vi "System@IncludeModule__Parameter.vi"(1 "ParamterIn":string) -> (0 "ParamterOut":string)   [LabVIEW 2020]
uses:
  MainFrame/Global.vi
panel:
  in  "Debug":string(combo)
  in  "Module":string(combo)
  in  "Confirm":bool
  # "System@IncludeModule $Module(,Debug)\nModule Directory is at MainPath\\ExternalModules\\$Module"
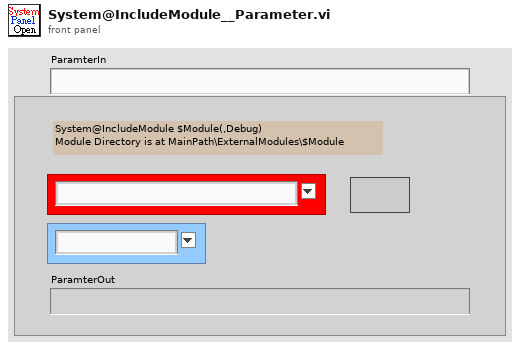
[diagram p1: front panel]
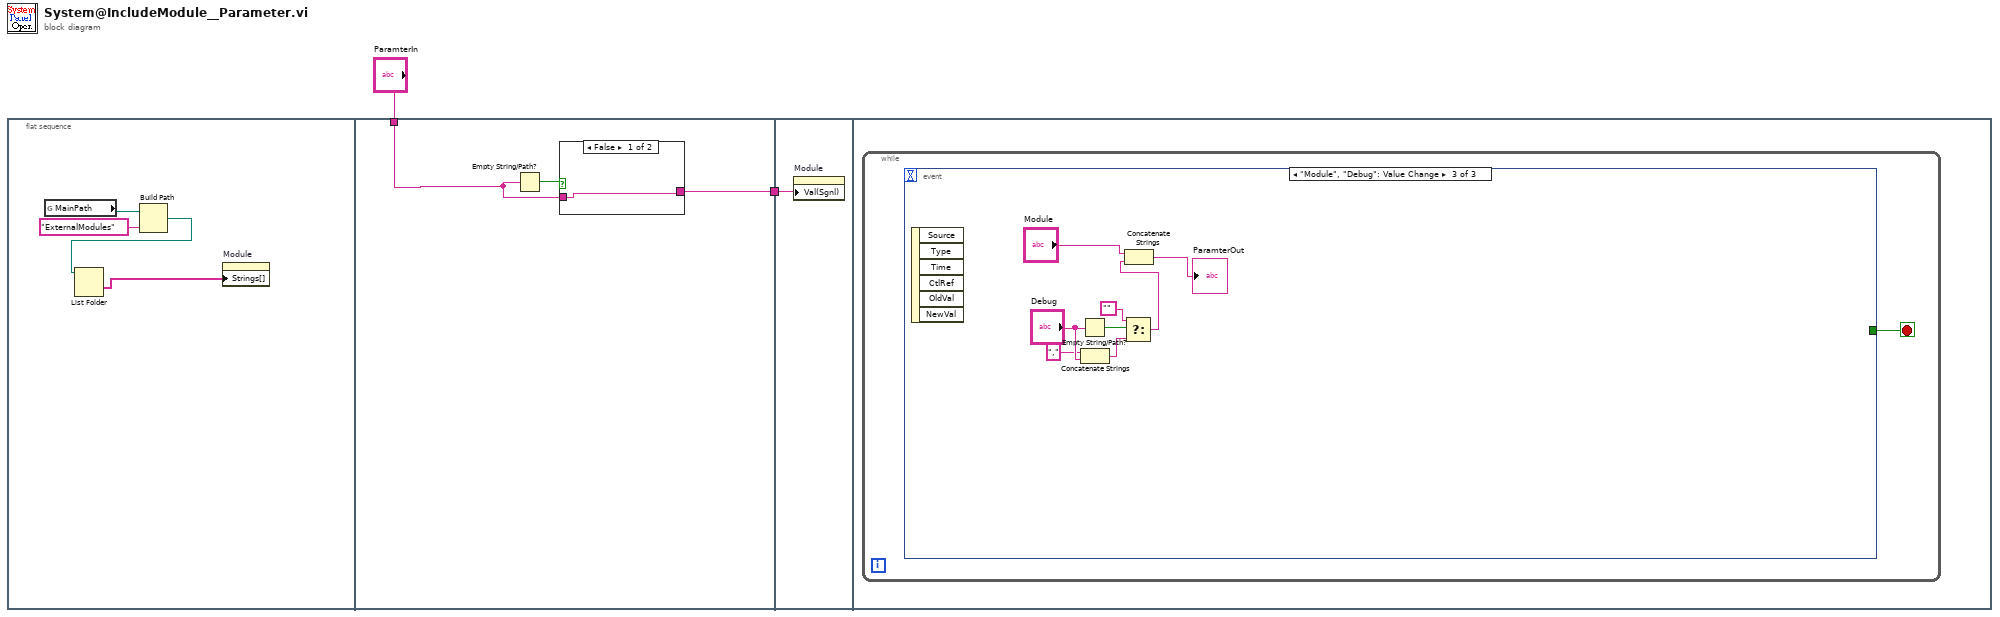
[diagram p0: block diagram]
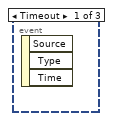
[diagram p3: hidden frame]
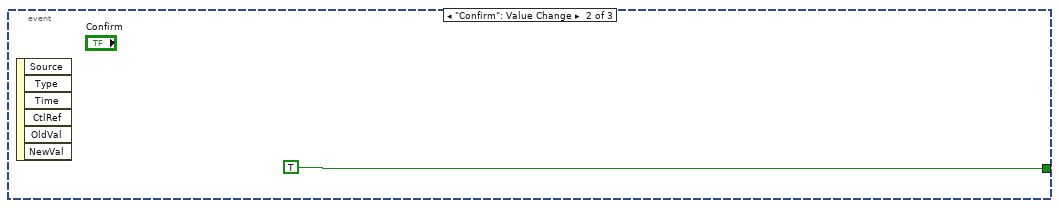
[diagram p4: hidden frame]
diagram:
  n1 = flat-sequence {
    tunnel: "ParamterIn" -> [w7]
    tunnel: [w8] -> w1
    tunnel: w1 -> [w12]
    frame #0 {
      n2 = global read "Global.vi" "MainPath"() -> (w6:path)
      n3 = Build Path(base path=w6, name or relative path="ExternalModules") -> (appended path=w4:path)
      n4 = List Folder(path=w4) -> (folder names=w3:string[])  [unwired: 3 in, 3 out]
      n5 = property on="Module" class="CmbBox"("Strings[]"=w3) -> ()  [unwired: 2 in, 2 out]
    }
    frame #1 {
      n6 = Empty String/Path?(string/path=w7) -> (empty?=w9:bool)
      n7 = case shown="False" w9 {
        tunnel: w7 -> [w10 w11]
        tunnel: [w10 w11] -> w8
        frame False {
        }
        frame True {
        }
      }
    }
    frame #2 {
      n8 = property on="Module" class="CmbBox"("Val(Sgnl)"=w12) -> ()  [unwired: 2 in, 2 out]
    }
    frame #3 {
      n9 = while {
        stop <- w13 stop-if-true
        n10 = event shown="[2] \"Module\", \"Debug\": Value Change" {
          selector: _ -> [_ _ _]
          dyn-events: _ -> [_ _ _]
          timeout: _ -> [_ _ _]
          tunnel: [_ TRUE _] -> w13
          event Timeout {
            n11 = event-data() -> ()  [unwired: 1 in, 3 out]
          }
          event "Confirm": Value Change {
            n12 = event-data() -> ()  [unwired: 1 in, 6 out]
          }
          event "Module", "Debug": Value Change {
            n13 = event-data() -> ()  [unwired: 1 in, 6 out]
            n14 = Empty String/Path?(string/path="Debug") -> (empty?=w22:bool)
            n15 = Concatenate Strings("," ("string"), "Debug") -> (w17:string)
            n16 = Select(t="", s=w22, f=w17) -> (s? t:f=w15:string)
            n17 = Concatenate Strings("Module", w15) -> (→"ParamterOut":string)
          }
        }
      }
    }
  }
